vi "培训1.vi"(6 "数值 3":dbl, 8 "数值 5":dbl) -> (4 "数值 6":dbl)   [LabVIEW 2019]
panel:
  out "数值 2":dbl
  out "数值 4":dbl
  in  "数值":dbl
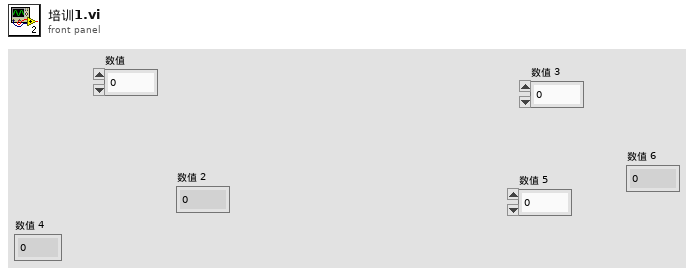
[diagram p1: front panel]
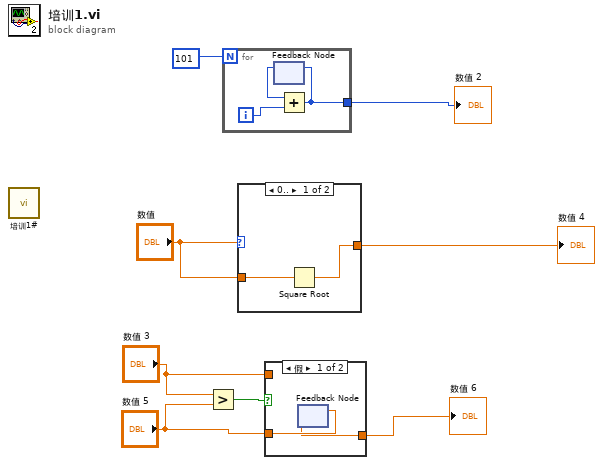
[diagram p0: block diagram]
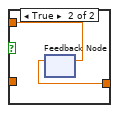
[diagram p2: hidden frame]
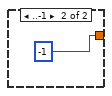
[diagram p3: hidden frame]
diagram:
  n1 = call "培训1#.vi"() -> ()  [unwired: 11 in, 1 out]
  n2 = Greater?(x="数值 3", y="数值 5") -> (0:w5:bool)
  n3 = for {
    N: 101 -> [_]
    tunnel: [w9] -> w1
    i -> [w11]
    n4 = feedback #1() -> (w10:i32)  [unwired: 1 in]
    n5 = Add(x=w10, y=w11) -> (x+y=w9:i32)
    n6 = feedback-in #1(w9) -> ()
  }
  "数值 2" <- w1
  n7 = case shown="0.." "数值" {
    tunnel: [w13 -1] -> w8
    tunnel: "数值" -> [w12 _]
    frame 0.. {
      n8 = Square Root(x=w12) -> (sqrt(x)=w13:dbl)
    }
    frame ..-1 {
    }
  }
  "数值 4" <- w8
  n9 = case shown="假" w5 {
    tunnel: "数值 3" -> [_ w18]
    tunnel: [w15 w17] -> w3
    tunnel: "数值 5" -> [w16 _]
    frame False {
      n10 = feedback-in #2(w16) -> ()
      n11 = feedback #2() -> (w15:dbl)  [unwired: 1 in]
    }
    frame True {
      n12 = feedback-in #3(w18) -> ()
      n13 = feedback #3() -> (w17:dbl)  [unwired: 1 in]
    }
  }
  "数值 6" <- w3
